vi "Destroy.vi"(8 "error in (no error)":errorcluster, 11 "Halt in":refnum<class "Halt.lvclass">) -> (0 "error out":errorcluster)   [LabVIEW 2017, in "Test Executive.lvlib" / "Halt.lvclass"]
uses:
  <vilib>/gpm_packages/@cs/test-executive/Source/Test Executive/Halt/Halt.lvclass
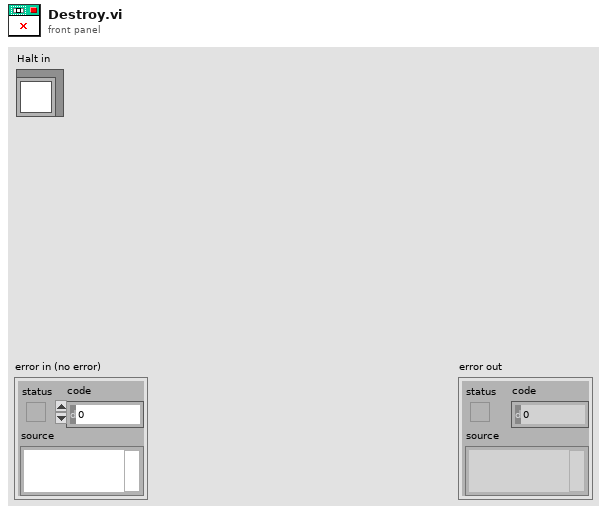
[diagram p1: front panel]
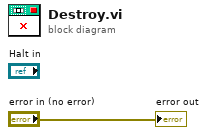
[diagram p0: block diagram]
diagram:
  "error out" <- "error in (no error)"
